vi "Recurse.vi"(6 "Error":errorcluster, 10 "ConcreteMessage":refnum<class "ConcreteMessage.lvclass">, 11 "Actor":refnum<class "Actor.lvclass">) -> (2 "ConcreteMessage":refnum<class "ConcreteMessage.lvclass">, 3 "Actor":refnum<class "Actor.lvclass">, 4 "Error":errorcluster)   [LabVIEW 2020, in "_Template.lvlib" / "MessageTemplate.lvlib" / "{{Name}}.lvlib"]
uses:
  {{Name}}.lvlib
  jettl/jettl/Actor/Actor.lvclass
  ConcreteMessage/ConcreteMessage.lvclass
panel:
  # "This front panel should not be manipulated."
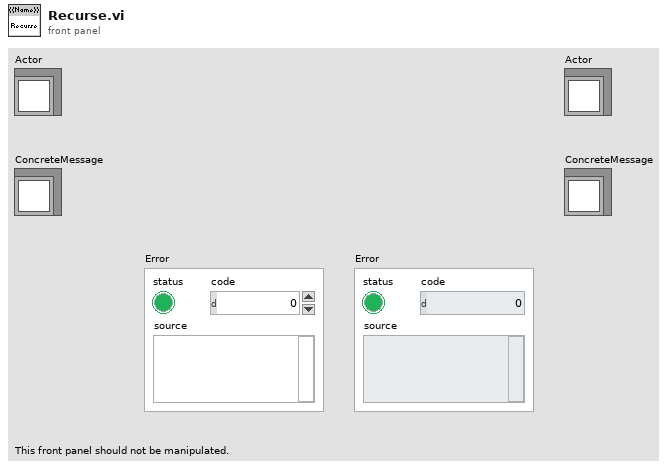
[diagram p1: front panel]
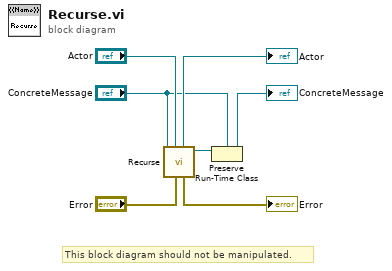
[diagram p0: block diagram]
diagram:
  # "This block diagram should not be manipulated."
  n1 = call-dynamic "Recurse.vi"("Error"="Error", "Actor"="Actor", "Message"="ConcreteMessage") -> ("Message"=w2:refnum<class "Message.lvclass">, "Error"=→"Error":errorcluster, "Actor"=→"Actor":refnum<class "Actor.lvclass">)  [unwired: 6 in]
  n2 = Preserve Run-Time Class(object in=w2, 2:"ConcreteMessage") -> (object out=→"ConcreteMessage":refnum<class "ConcreteMessage.lvclass">)  [unwired: 1 in, 1 out]
